vi "RT_NetStreams.vi"() -> ()   [LabVIEW 2019]
panel:
  out "error out":errorcluster
  out "Waveform Graph":dbl[](graph)
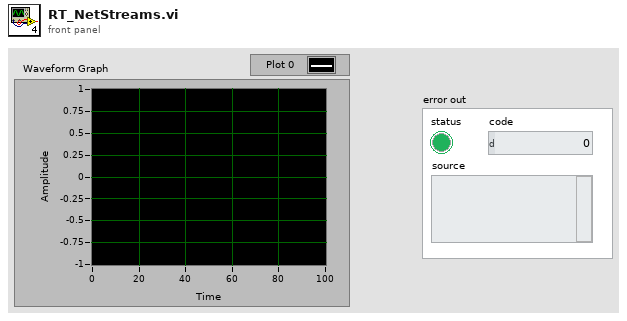
[diagram p1: front panel]
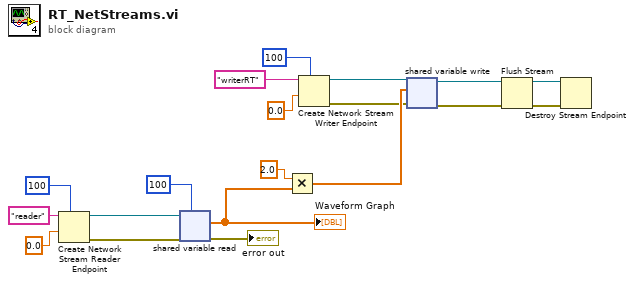
[diagram p0: block diagram]
diagram:
  n1 = Create Network Stream Reader Endpoint(7:100 ("reader buffer size"), 9:0.0 ("sin(x)"), 11:"reader" ("reader name")) -> (0:w14:errorcluster, 3:w15:refnum<k21>)  [unwired: 4 in]
  n2 = shared-variable-read(w15, w14, 100 ("# elements")) -> (→"error out":errorcluster, w11:dbl[])  [unwired: 1 in, 2 out]
  "Waveform Graph" <- w11
  n3 = Multiply(x=2.0, y=w11) -> (x*y=w19:dbl[])
  n4 = Create Network Stream Writer Endpoint(7:100 ("writer buffer size"), 9:0.0 ("sin(x)"), 11:"writerRT" ("writer name")) -> (0:w6:errorcluster, 3:w7:refnum<k21>)  [unwired: 4 in]
  n5 = shared-variable-write(w7, w6, w19) -> (w4:refnum<k21>, w5:errorcluster)  [unwired: 1 in, 1 out]
  n6 = Flush Stream(8:w5, 11:w4) -> (0:w9:errorcluster, 3:w8:refnum<k21>)  [unwired: 2 in, 1 out]
  n7 = Destroy Stream Endpoint(8:w9, 11:w8) -> ()  [unwired: 1 out]
